vi "Comm EXE Get EXE Path.vi"(8 "error in (no error)":errorcluster, 11 "niDTS Comm EXE in":refnum<class "niDTS Comm EXE.lvclass">) -> (0 "error out":errorcluster, 2 "EXE Path":path, 3 "niDTS Comm EXE out":refnum<class "niDTS Comm EXE.lvclass">)   [LabVIEW 2015, in "niDTS CommLib.lvlib" / "niDTS Comm EXE.lvclass"]
uses:
  niDTS Comm EXE.lvclass
  niDTS Comm EXE.lvclass/niDTS Comm EXE.ctl
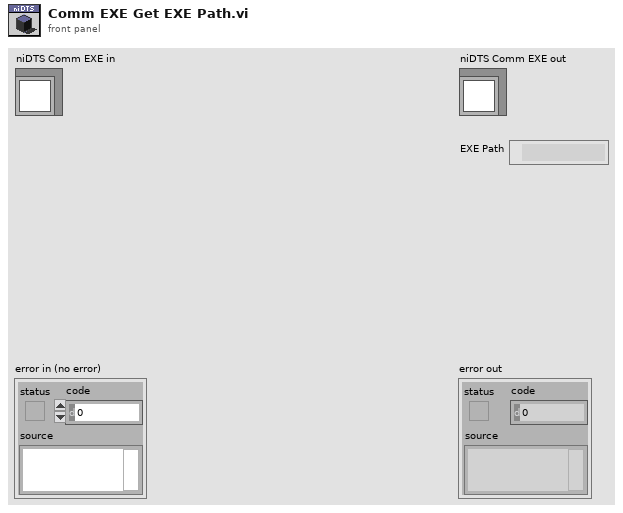
[diagram p1: front panel]
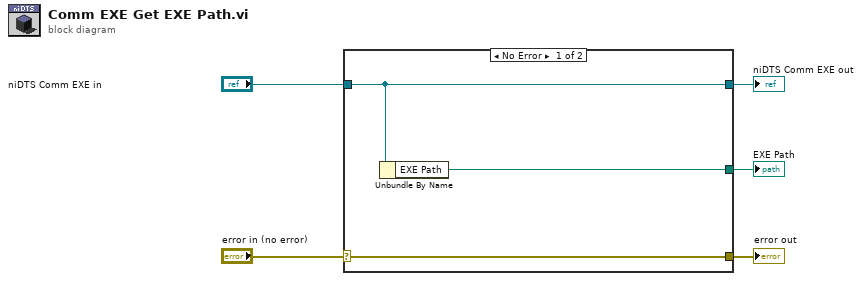
[diagram p0: block diagram]
diagram:
  n1 = case shown="No Error" "error in (no error)" {
    selector: "error in (no error)" -> [w8 w9]
    tunnel: [w8 w9] -> w4
    tunnel: [w7 w10] -> w2
    tunnel: "niDTS Comm EXE in" -> [w7 w10]
    tunnel: [w6 _] -> w1
    frame No Error {
      n2 = Unbundle By Name(w7) -> ("EXE Path"=w6:path)
    }
    frame Error {
    }
  }
  "error out" <- w4
  "niDTS Comm EXE out" <- w2
  "EXE Path" <- w1
